vi "write_params.vi"(8 "error in (no error)":errorcluster, 10 "params":T1={"n_estimators"=100.0, "criterion"="gini", "max_depth"={"max_depth_type"="None", "max_depth_int"=0.0}, "min_samples_split"=2.0, "min_samples_leaf"=1.0, "min_weight_fraction_leaf"=0.0, "max_features"={"max_features_type"="auto", "max_features_int"=0.0, "max_features_float"=0.0}, "max_leaf_nodes"={"max_leaf_nodes_type"="None", "max_leaf_nodes_int"=100.0}, "min_impurity_decrease"=0.0, "bootstrap"=TRUE, "oob_score"=FALSE, "n_jobs"=1.0, "random_state"=0.0, "verbose"=0.0, "warm_start"=FALSE, "class_weight"={"class_weight_type"="None", "class_weight_dict"="{0:1.1, 2:1.5, 2:0.6}"}, "ccp_alpha"=0.0, "max_samples"={"max_samples_type"="None", "max_samples_int"=0.0, "max_samples_float"=0.0}}, 11 "RandomForestClassifier in":refnum<class "RandomForestClassifier.lvclass">) -> (0 "error out":errorcluster, 3 "RandomForestClassifier out":refnum<class "RandomForestClassifier.lvclass">)   [LabVIEW 2020, in "RandomForestClassifier.lvclass"]
uses:
  RandomForestClassifier.lvclass
  Controls/random_forest_classifier_params.ctl
  RandomForestClassifier.lvclass/RandomForestClassifier.ctl
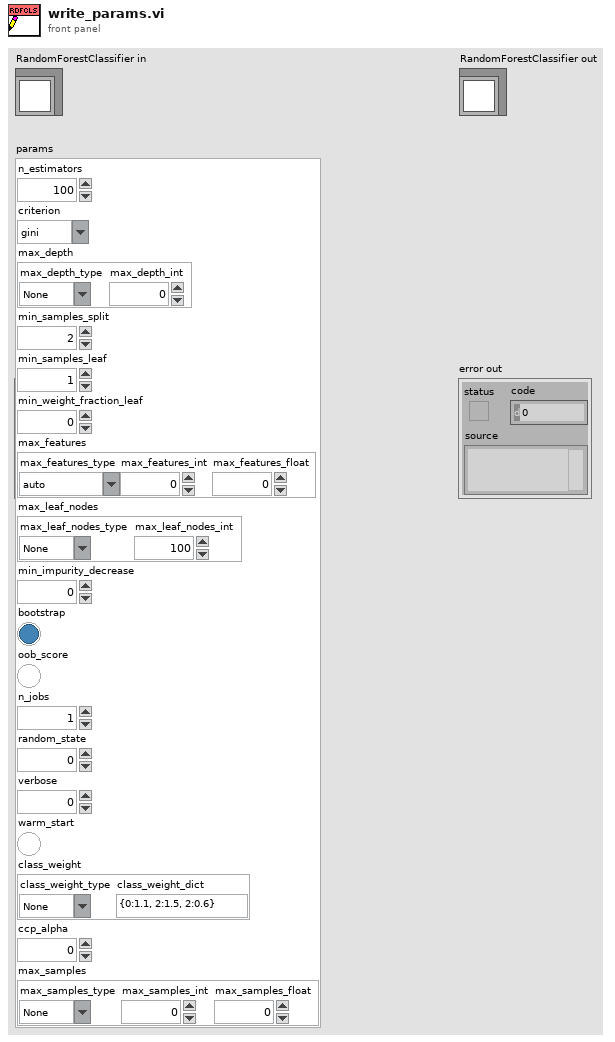
[diagram p1: front panel]
types:
  T1 = typedef "random_forest_classifier_params.ctl" = cluster{"n_estimators":dbl, "criterion":string, "max_depth":cluster{"max_depth_type":string, "max_depth_int":dbl}, "min_samples_split":dbl, "min_samples_leaf":dbl, "min_weight_fraction_leaf":dbl, "max_features":cluster{"max_features_type":string, "max_features_int":dbl, "max_features_float":dbl}, "max_leaf_nodes":cluster{"max_leaf_nodes_type":string, "max_leaf_nodes_int":dbl}, "min_impurity_decrease":dbl, "bootstrap":bool, "oob_score":bool, "n_jobs":dbl, "random_state":dbl, "verbose":dbl, "warm_start":bool, "class_weight":cluster{"class_weight_type":string, "class_weight_dict":string}, "ccp_alpha":dbl, "max_samples":cluster{"max_samples_type":string, "max_samples_int":dbl, "max_samples_float":dbl}}
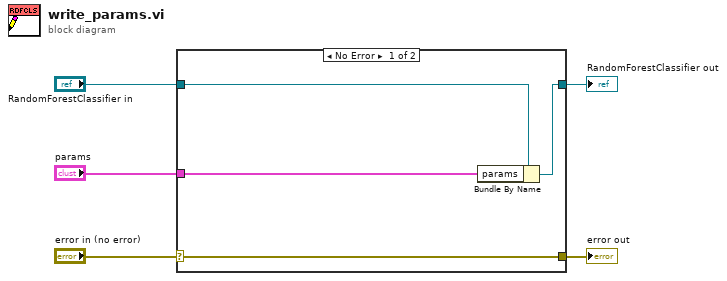
[diagram p0: block diagram]
diagram:
  n1 = case shown="No Error" "error in (no error)" {
    selector: "error in (no error)" -> [w9 w10]
    tunnel: [w9 w10] -> w4
    tunnel: [w7 w11] -> w2
    tunnel: "RandomForestClassifier in" -> [w8 w11]
    tunnel: "params" -> [w6 _]
    frame No Error {
      n2 = Bundle By Name(cluster=w8, "params"=w6) -> (w7:refnum<class "RandomForestClassifier.lvclass">)
    }
    frame Error {
    }
  }
  "error out" <- w4
  "RandomForestClassifier out" <- w2
